vi "PresetServiceData.vi"(5 "Data":i16=500 min=-2 max=255 step=1, 6 "Enable":bool, 7 "Command":u16, 8 "error in":errorcluster, 10 "Cluster in":T1, 11 "VISA Refnum in":refnum<visa-resource-name>) -> (0 "error out":errorcluster, 2 "Cluster Out":T1, 3 "VISA resource name out":refnum<visa-resource-name>)   [LabVIEW 2020]
uses:
  91005176-02cb-46eb-9406-a8501dd599b0.vi
  9dcd1051-5816-47e2-ae31-a75755c11cd0.vi
  9dcd1051-5816-47e2-ae31-a75755c11cd0.vi/393b2312-c94a-42b8-a7f2-b1ce51657457.vi
  <vilib>/NI Modbus.llb/MB Serial Master Query (poly).vi
  <vilib>/NI Modbus.llb/MB Serial Master Query Write Single Register (poly).vi
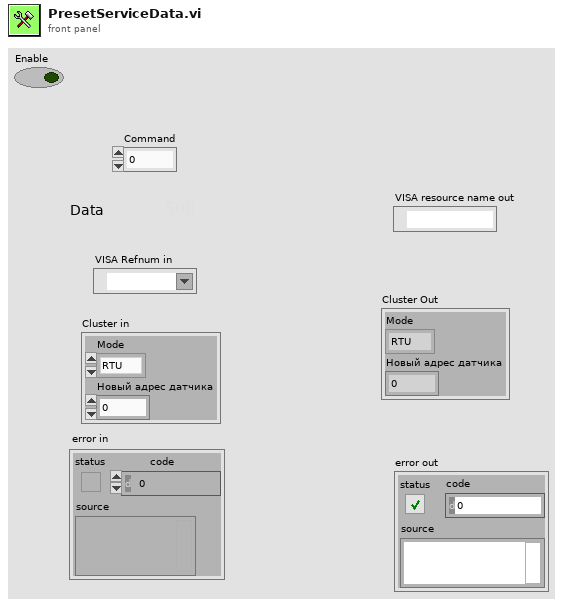
[diagram p1: front panel]
types:
  T1 = cluster{"Mode":enum16{"RTU", "ASCII"}, "Новый адрес датчика":u16}
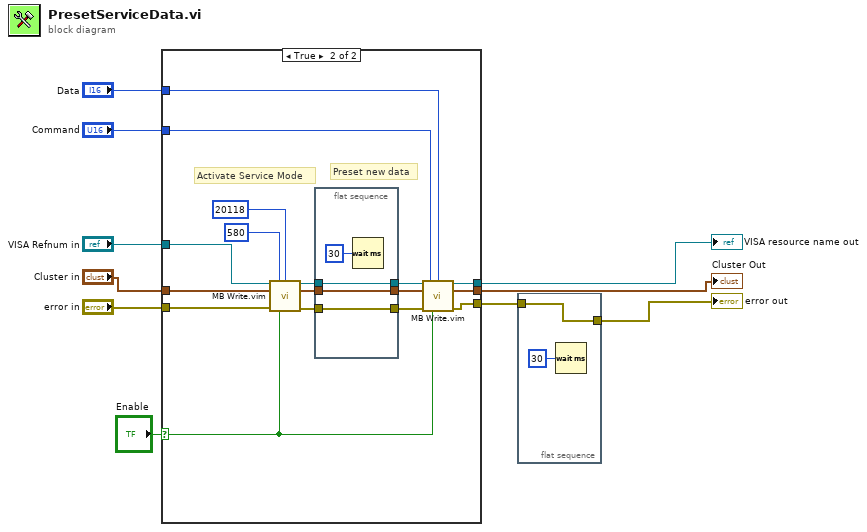
[diagram p0: block diagram]
diagram:
  n1 = case shown="True" "Enable" {
    selector: "Enable" -> [_ w14]
    tunnel: "VISA Refnum in" -> [w13 w30]
    tunnel: "Cluster in" -> [w12 w29]
    tunnel: "error in" -> [w11 w28]
    tunnel: "Command" -> [_ w19]
    tunnel: "Data" -> [_ w18]
    tunnel: [w13 w17] -> w5
    tunnel: [w12 w16] -> w4
    tunnel: [w11 w15] -> w3
    frame False {
    }
    frame True {
      # "Preset new data"
      # "Activate Service Mode"
      n2 = call "MB Write.vim"("VISA Refnum in"=w30, "Command"=u16 580, "Data"=u16 20118, "Cluster"=w29, "error in"=w28, "Enable"=w14) -> ("VISA out"=w24:refnum<visa-resource-name>, "Cluster Out"=w22:T1, "error out"=w27:errorcluster)  [unwired: 7 in]
      n3 = flat-sequence {
        tunnel: w27 -> [w34]
        tunnel: [w34] -> w26
        tunnel: [w32] -> w25
        tunnel: w24 -> [w32]
        tunnel: [w31] -> w23
        tunnel: w22 -> [w31]
        frame #0 {
          n4 = Wait (ms)(milliseconds to wait=u32 30) -> ()  [unwired: 1 out]
        }
      }
      n5 = call "MB Write.vim"("VISA Refnum in"=w25, "Command"=w19, "Data"=w18, "Cluster"=w23, "error in"=w26, "Enable"=w14) -> ("VISA out"=w17:refnum<visa-resource-name>, "Cluster Out"=w16:T1, "error out"=w15:errorcluster)  [unwired: 7 in]
    }
  }
  "VISA resource name out" <- w5
  "Cluster Out" <- w4
  n6 = flat-sequence {
    tunnel: w3 -> [w35]
    tunnel: [w35] -> w2
    frame #0 {
      n7 = Wait (ms)(milliseconds to wait=u32 30) -> ()  [unwired: 1 out]
    }
  }
  "error out" <- w2
